vi "Stop Streaming Waveforms.vi"(8 "error in (no error)":errorcluster, 10 "WaveformStreamSpecifications":T1[](array[typedef]), 11 "WaveformStreaming in":T2) -> (0 "error out":errorcluster, 3 "WaveformStreaming out":T2)   [LabVIEW 2020, in "NI_VS Waveform Streaming Interface.lvlib"]
doc: "Stops streaming the specified waveforms to the VeriStand Gateway."
uses:
  <vilib>/NI VeriStand/Execution/WaveformStreaming/NI_VS Waveform Streaming Interface.lvlib
  <vilib>/NI VeriStand/Execution/WaveformStreaming/WaveformStreamingAPI.ctl
  NationalInstruments.VeriStand.ClientAPI
  <vilib>/NI VeriStand/Execution/WaveformStreaming/WaveformStreamSpecification.ctl
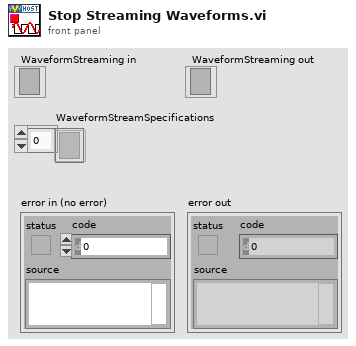
[diagram p1: front panel]
types:
  T1 = typedef "NI_VS Waveform Streaming Interface.lvlib/WaveformStreamSpecification.ctl" = refnum<k24>
  T2 = typedef "NI_VS Waveform Streaming Interface.lvlib/WaveformStreamingAPI.ctl" = refnum<k24>
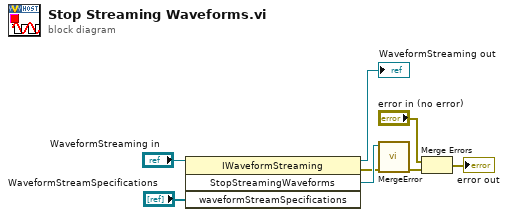
[diagram p0: block diagram]
diagram:
  n1 = invoke class="IWaveformStreaming" method="StopStreamingWaveforms"(reference="WaveformStreaming in", "waveformStreamSpecifications"="WaveformStreamSpecifications") -> (reference out=→"WaveformStreaming out":T2, error out=w2:errorcluster, "StopStreamingWaveforms"=w3:refnum<k24>)  [unwired: 2 in, 1 out]
  n2 = call <vilib>:"MergeError.vi"("error in (no error)"=w2, "Error"=w3) -> ("error out"=w1:errorcluster)  [unwired: 9 in]
  n3 = Merge Errors("error in (no error)", w1) -> (→"error out":errorcluster)
